vi "SaveScoreImages.vi"(3 "Color Table":u32[](array[colorbox])=[0, 0, 65793, 131586, 197379, 263172, 328965, 394758, 460551, 526344, 592137, 657930, 723723, 789516, 855309, 921102, 986895, 1052688, 1118481, 1184274, 1250067, 1315860, 1381653, 1447446, 1513239, 1579032, 1644825, 1710618, 1776411, 1842204, 1907997, 1973790, 2039583, 2105376, 2171169, 2236962, 2302755, 2368548, 2434341, 2500134, 2565927, 2631720, 2697513, 2763306, 2829099, 2894892, 2960685, 3026478, 3092271, 3158064, 3223857, 3289650, 3355443, 3421236, 3487029, 3552822, 3618615, 3684408, 3750201, 3815994, 3881787, 3947580, 4013373, 4079166, 4144959, 4210752, 4276545, 4342338, 4408131, 4473924, 4539717, 4605510, 4671303, 4737096, 4802889, 4868682, 4934475, 5000268, 5066061, 5131854, 5197647, 5263440, 5329233, 5395026, 5460819, 5526612, 5592405, 5658198, 5723991, 5789784, 5855577, 5921370, 5987163, 6052956, 6118749, 6184542, 6250335, 6316128, 6381921, 6447714, 6513507, 6579300, 6645093, 6710886, 6776679, 6842472, 6908265, 6974058, 7039851, 7105644, 7171437, 7237230, 7303023, 7368816, 7434609, 7500402, 7566195, 7631988, 7697781, 7763574, 7829367, 7895160, 7960953, 8026746, 8092539, 8158332, 8224125, 8289918, 8355711, 8421504, 8487297, 8553090, 8618883, 8684676, 8750469, 8816262, 8882055, 8947848, 9013641, 9079434, 9145227, 9211020, 9276813, 9342606, 9408399, 9474192, 9539985, 9605778, 9671571, 9737364, 9803157, 9868950, 9934743, 10000536, 10066329, 10132122, 10197915, 10263708, 10329501, 10395294, 10461087, 10526880, 10592673, 10658466, 10724259, 10790052, 10855845, 10921638, 10987431, 11053224, 11119017, 11184810, 11250603, 11316396, 11382189, 11447982, 11513775, 11579568, 11645361, 11711154, 11776947, 11842740, 11908533, 11974326, 12040119, 12105912, 12171705, 12237498, 12303291, 12369084, 12434877, 12500670, 12566463, 12632256, 12698049, 12763842, 12829635, 12895428, 12961221, 13027014, 13092807, 13158600, 13224393, 13290186, 13355979, 13421772, 13487565, 13553358, 13619151, 13684944, 13750737, 13816530, 13882323, 13948116, 14013909, 14079702, 14145495, 14211288, 14277081, 14342874, 14408667, 14474460, 14540253, 14606046, 14671839, 14737632, 14803425, 14869218, 14935011, 15000804, 15066597, 15132390, 15198183, 15263976, 15329769, 15395562, 15461355, 15527148, 15592941, 15658734, 15724527, 15790320, 15856113, 15921906, 15987699, 16053492, 16119285, 16185078, 16250871, 16316664, 16382457, 6352640, 12058434, 16770066, 16758546, 16711731], 5 "Save Directory":path, 7 "FileName":string, 8 "Colored Score":dbl[][](array[numeric]), 9 "colored Int":dbl[][](array[numeric]), 10 "Colored MB":dbl[][](array[numeric]), 11 "Scaled Score":dbl[][](array[numeric])) -> ()   [LabVIEW 2022 SP3]
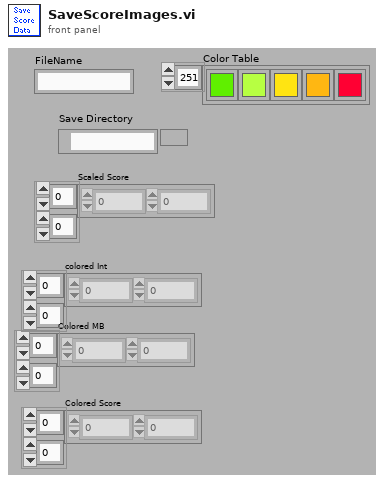
[diagram p1: front panel]
types:
  T1 = typedef "imagedata.ctl" = cluster{"image type":i32, "image depth":i32, "image":u8[], "mask":u8[], "colors":u32[], "Rectangle":cluster{"left":i16, "top":i16, "right":i16, "bottom":i16}}
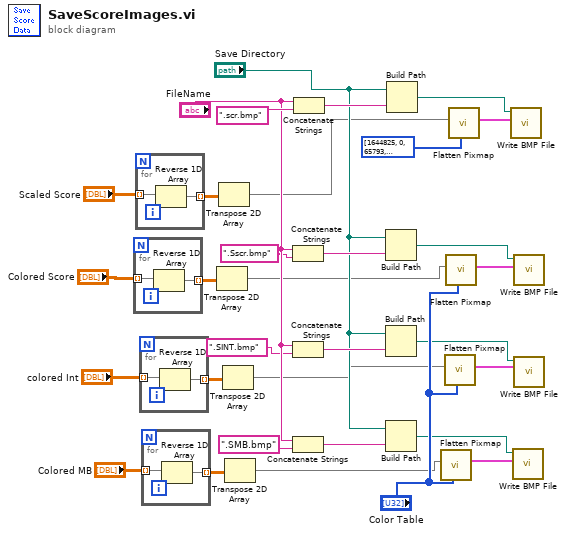
[diagram p0: block diagram]
diagram:
  n1 = for {
    tunnel: "Colored Score" -> [w34] mode=indexing
    tunnel: [w33] -> w5 mode=indexing
    n2 = Reverse 1D Array(array=w34) -> (reversed array=w33:dbl[])
  }
  n3 = for {
    tunnel: "Scaled Score" -> [w36] mode=indexing
    tunnel: [w35] -> w6 mode=indexing
    n4 = Reverse 1D Array(array=w36) -> (reversed array=w35:dbl[])
  }
  n5 = for {
    tunnel: "colored Int" -> [w38] mode=indexing
    tunnel: [w37] -> w4 mode=indexing
    n6 = Reverse 1D Array(array=w38) -> (reversed array=w37:dbl[])
  }
  n7 = for {
    tunnel: "Colored MB" -> [w40] mode=indexing
    tunnel: [w39] -> w10 mode=indexing
    n8 = Reverse 1D Array(array=w40) -> (reversed array=w39:dbl[])
  }
  n9 = Transpose 2D Array(2D array=w5) -> (transposed array=w2:dbl[][])
  n10 = Transpose 2D Array(2D array=w6) -> (transposed array=w1:dbl[][])
  n11 = Transpose 2D Array(2D array=w4) -> (transposed array=w3:dbl[][])
  n12 = Transpose 2D Array(2D array=w10) -> (transposed array=w12:dbl[][])
  n13 = Concatenate Strings("FileName", ".Sscr.bmp") -> (w30:string)
  n14 = Concatenate Strings("FileName", ".SINT.bmp") -> (w29:string)
  n15 = Concatenate Strings("FileName", ".SMB.bmp") -> (w28:string)
  n16 = Concatenate Strings("FileName", ".scr.bmp") -> (w31:string)
  n17 = Build Path(base path="Save Directory", name or relative path=w30) -> (appended path=w22:path)
  n18 = Build Path(base path="Save Directory", name or relative path=w29) -> (appended path=w21:path)
  n19 = Build Path(base path="Save Directory", name or relative path=w28) -> (appended path=w20:path)
  n20 = Build Path(base path="Save Directory", name or relative path=w31) -> (appended path=w19:path)
  n21 = call <vilib>:"Flatten Pixmap.vi"("colors"="Color Table", "8-bit pixmap"=w12) -> ("image data"=w24:T1)  [unwired: 4 in, 5 out]
  n22 = call <vilib>:"Flatten Pixmap.vi"("colors"="Color Table", "8-bit pixmap"=w3) -> ("image data"=w25:T1)  [unwired: 4 in, 5 out]
  n23 = call <vilib>:"Flatten Pixmap.vi"("colors"="Color Table", "8-bit pixmap"=w2) -> ("image data"=w26:T1)  [unwired: 4 in, 5 out]
  n24 = call <vilib>:"Flatten Pixmap.vi"("colors"=u32[] [1644825, 0, 65793, 131586, 197379, 263172, 328965, 394758, 460551, 526344, 592137, 657930, 723723, 789516, 855309, 921102, 986895, 1052688, 1118481, 1184274, 1250067, 1315860, 1381653, 1447446, 1513239, 1579032, 1644825, 1710618, 1776411, 1842204, 1907997, 1973790, 2039583, 2105376, 2171169, 2236962, 2302755, 2368548, 2434341, 2500134, 2565927, 2631720, 2697513, 2763306, 2829099, 2894892, 2960685, 3026478, 3092271, 3158064, 3223857, 3289650, 3355443, 3421236, 3487029, 3552822, 3618615, 3684408, 3750201, 3815994, 3881787, 3947580, 4013373, 4079166, 4144959, 4210752, 4276545, 4342338, 4408131, 4473924, 4539717, 4605510, 4671303, 4737096, 4802889, 4868682, 4934475, 5000268, 5066061, 5131854, 5197647, 5263440, 5329233, 5395026, 5460819, 5526612, 5592405, 5658198, 5723991, 5789784, 5855577, 5921370, 5987163, 6052956, 6118749, 6184542, 6250335, 6316128, 6381921, 6447714, 6513507, 6579300, 6645093, 6710886, 6776679, 6842472, 6908265, 6974058, 7039851, 7105644, 7171437, 7237230, 7303023, 7368816, 7434609, 7500402, 7566195, 7631988, 7697781, 7763574, 7829367, 7895160, 7960953, 8026746, 8092539, 8158332, 8224125, 8289918, 8355711, 8421504, 8487297, 8553090, 8618883, 8684676, 8750469, 8816262, 8882055, 8947848, 9013641, 9079434, 9145227, 9211020, 9276813, 9342606, 9408399, 9474192, 9539985, 9605778, 9671571, 9737364, 9803157, 9868950, 9934743, 10000536, 10066329, 10132122, 10197915, 10263708, 10329501, 10395294, 10461087, 10526880, 10592673, 10658466, 10724259, 10790052, 10855845, 10921638, 10987431, 11053224, 11119017, 11184810, 11250603, 11316396, 11382189, 11447982, 11513775, 11579568, 11645361, 11711154, 11776947, 11842740, 11908533, 11974326, 12040119, 12105912, 12171705, 12237498, 12303291, 12369084, 12434877, 12500670, 12566463, 12632256, 12698049, 12763842, 12829635, 12895428, 12961221, 13027014, 13092807, 13158600, 13224393, 13290186, 13355979, 13421772, 13487565, 13553358, 13619151, 13684944, 13750737, 13816530, 13882323, 13948116, 14013909, 14079702, 14145495, 14211288, 14277081, 14342874, 14408667, 14474460, 14540253, 14606046, 14671839, 14737632, 14803425, 14869218, 14935011, 15000804, 15066597, 15132390, 15198183, 15263976, 15329769, 15395562, 15461355, 15527148, 15592941, 15658734, 15724527, 15790320, 15856113, 15921906, 15987699, 16053492, 16119285, 16185078, 16250871, 16316664, 16382457, 16448250, 16514043, 16579836, 16645629, 16711680] ("Color Table"), "8-bit pixmap"=w1) -> ("image data"=w27:T1)  [unwired: 4 in, 5 out]
  n25 = call <vilib>:"Write BMP File.vi"("image data"=w27, "path to BMP file"=w19) -> ()  [unwired: 1 in, 9 out]
  n26 = call <vilib>:"Write BMP File.vi"("image data"=w24, "path to BMP file"=w20) -> ()  [unwired: 1 in, 9 out]
  n27 = call <vilib>:"Write BMP File.vi"("image data"=w26, "path to BMP file"=w22) -> ()  [unwired: 1 in, 9 out]
  n28 = call <vilib>:"Write BMP File.vi"("image data"=w25, "path to BMP file"=w21) -> ()  [unwired: 1 in, 9 out]
